vi "test_getPhoton.vi"() -> ()   [LabVIEW 2018, in "Photon Filtering.lvlib"]
uses:
  Photon Filtering.lvlib
  <vilib>/Analysis/baseanly.llb/Real Outer Product.vi
  <vilib>/Analysis/Matrix/Numeric/Conversions/Matrix To Array - RM.vi
  <vilib>/Analysis/NI_AALBase.lvlib
  <vilib>/Analysis/Matrix/NI_Matrix.lvlib
panel:
  in  "fft cluster":T1
  in  "filtered int/phase":bool=TRUE
  in  "Mask ON":bool
  in  "FFT int/phase":bool=TRUE
  in  "Filter on/off":bool=TRUE
  out "FFT":dbl[][](graph)
  out "filtered  FFT":dbl[][](graph)
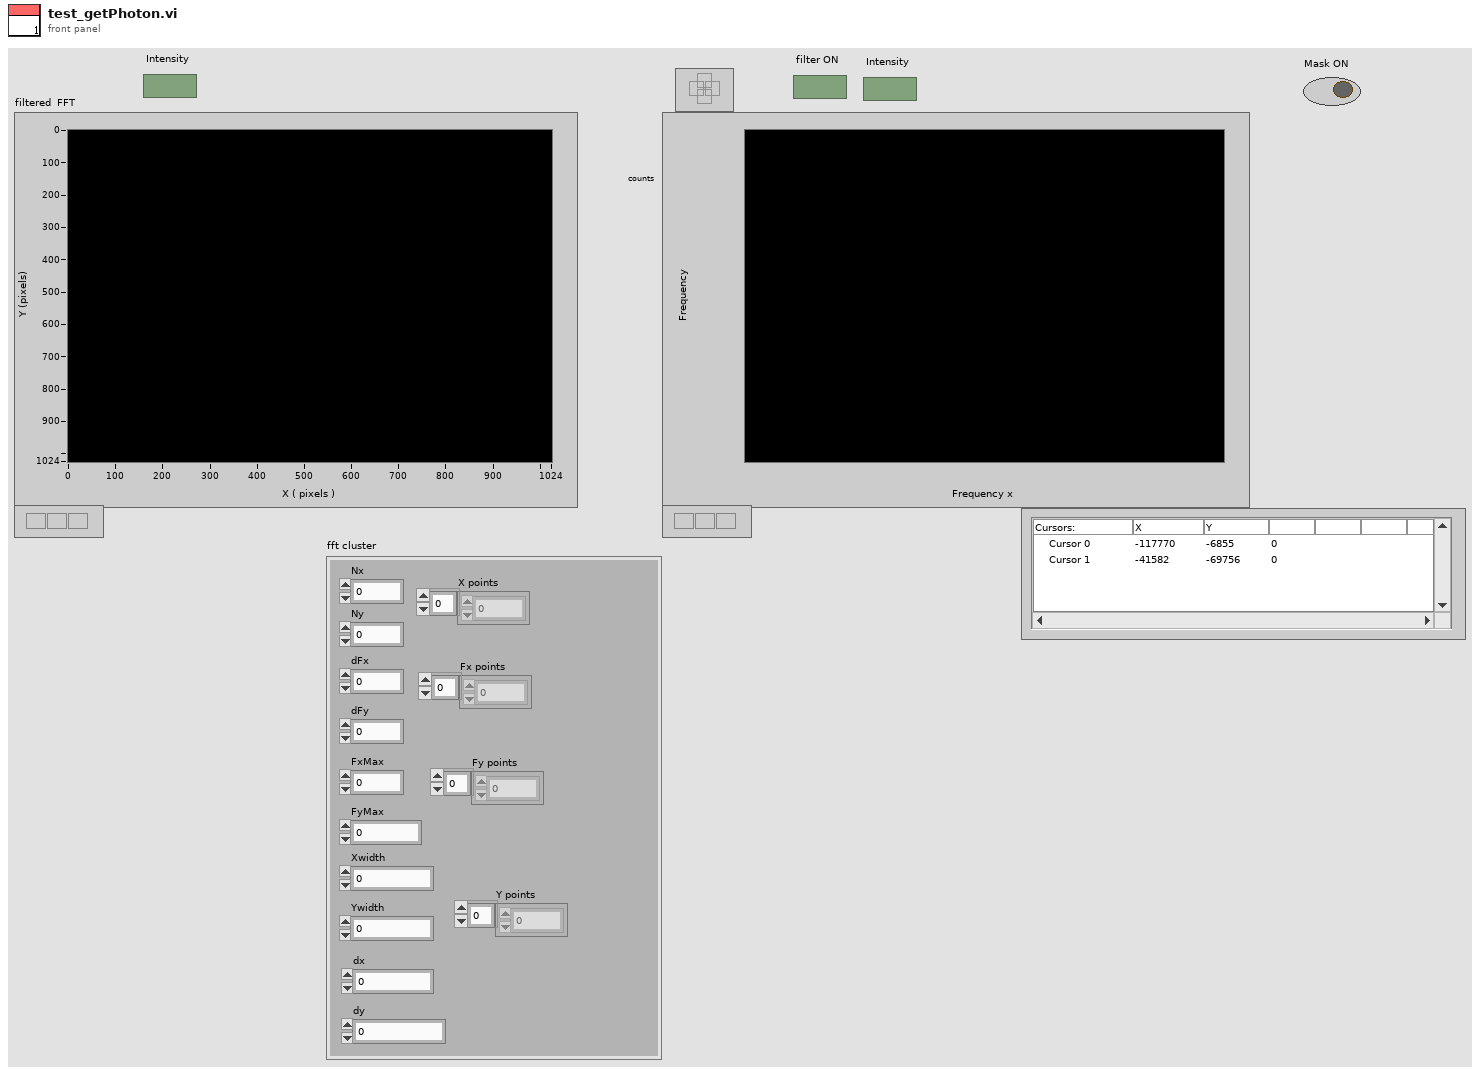
[diagram p1: front panel]
types:
  T1 = cluster{"dFx":dbl, "dFy":dbl, "Nx":i32, "Ny":i32, "FxMax":dbl, "FyMax":dbl, "Xwidth":dbl, "Ywidth":dbl, "dx":dbl, "dy":dbl, "Fx points":dbl[], "X points":dbl[], "Y points":dbl[], "Fy points":dbl[]}
  T2 = typedef "NI_Matrix.lvlib/RealMatrix.ctl" = dbl[][]
  T3 = cluster{"Filter on/off":bool, "filtered int/phase":bool, "Mask ON":bool, "FFT int/phase":bool}
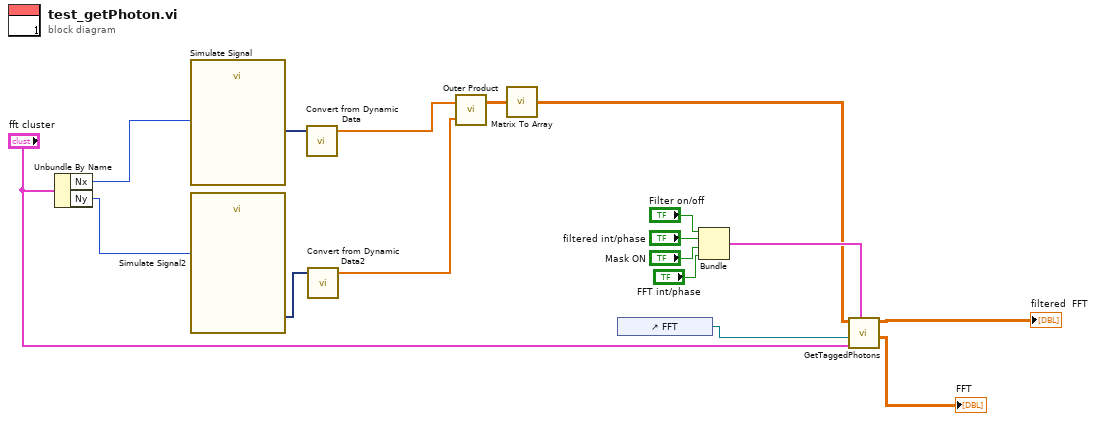
[diagram p0: block diagram]
diagram:
  n1 = Unbundle By Name("fft cluster") -> ("Nx"=w7:i32, "Ny"=w4:i32)
  n2 = call "Simulate Signal"("Seed Number"=w7) -> ("Sine with Inverse F Noise"=w8:dynamicdata)  [unwired: 13 in, 1 out]
  n3 = call "Simulate Signal2"("Seed Number"=w4) -> ("Sine with Inverse F Noise"=w3:dynamicdata)  [unwired: 13 in, 1 out]
  n4 = call "Convert from Dynamic Data"("Dynamic Data Type"=w8) -> ("Array"=w9:dbl[])  [unwired: 3 in]
  n5 = call "Convert from Dynamic Data2"("Dynamic Data Type"=w3) -> ("Array"=w2:dbl[])  [unwired: 3 in]
  n6 = call-poly <vilib>:"Outer Product.vi"("Y Vector"=w2, "X Vector"=w9) -> ("Outer Product"=w10:T2)  [unwired: 1 out]
  n7 = call-poly <vilib>:"Matrix To Array.vi"("Real Matrix"=w10) -> ("Real 2D Array"=w6:dbl[][])
  n8 = control-ref of="FFT"() -> (w12:refnum<vi>)
  n9 = Bundle("Filter on/off"="Filter on/off", "filtered int/phase"="filtered int/phase", "Mask ON"="Mask ON", "FFT int/phase"="FFT int/phase") -> (w13:T3)  [unwired: 1 in]
  n10 = call "GetTaggedPhotons.vi"("screen status"=w13, "fft cluster"="fft cluster", "FFT reference"=w12, "double precision float"=w6) -> ("FFT modulous"=→"FFT":dbl[][], "tagged photons"=→"filtered  FFT":dbl[][])  [unwired: 4 in, 2 out]
